vi "Init.vi"(5 "Bus In":refnum<class "Bus.lvclass">, 7 "Cluster":T1, 8 "error in (no error)":errorcluster, 9 "Init or Array":bool, 10 "Array":dbl[](array[numeric]), 11 "No-Op in":refnum<class "No-Op Output.lvclass">) -> (0 "error out":errorcluster, 2 "Bus Out":refnum<class "Bus.lvclass">, 3 "No-Op out":refnum<class "No-Op Output.lvclass">)   [LabVIEW 2024, in "No-Op Output.lvclass"]
uses:
  No-Op Output.lvclass
  Scaling/Scaling.lvclass
  Bus/Bus.lvclass
  No-Op Output.lvclass/No-Op Output.ctl
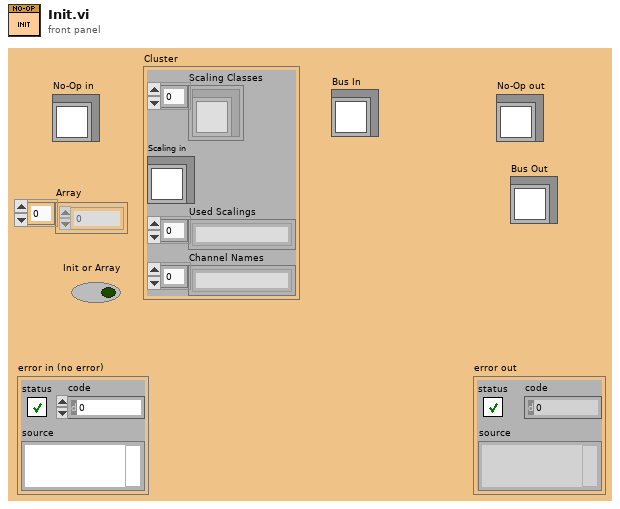
[diagram p1: front panel]
types:
  T1 = cluster{"Scaling Classes":refnum<class "Scaling.lvclass">[], "Scaling in":refnum<class "Scaling.lvclass">, "Used Scalings":string[], "Channel Names":string[]}
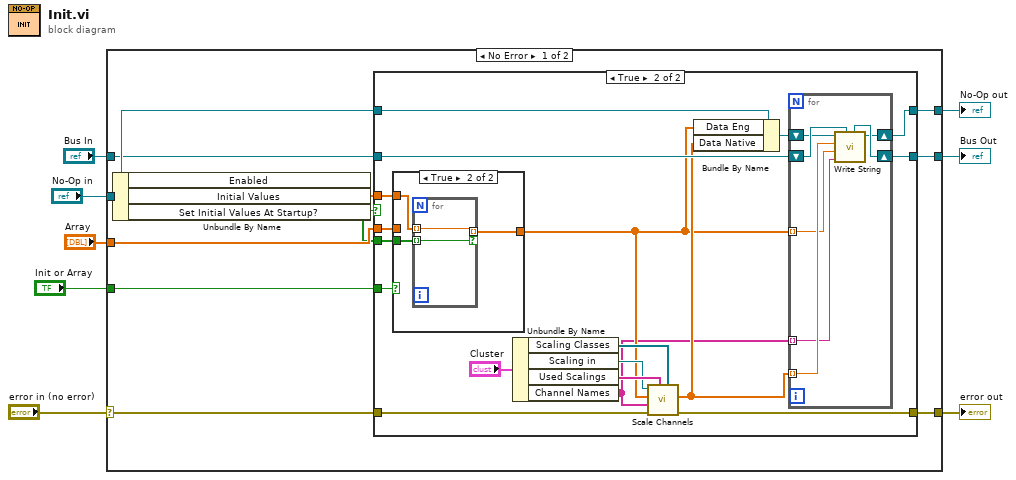
[diagram p0: block diagram]
diagram:
  n1 = case shown="No Error" "error in (no error)" {
    selector: "error in (no error)" -> [w16 w59]
    tunnel: [w15 w59] -> w7
    tunnel: [w12 w60] -> w6
    tunnel: "No-Op in" -> [w19 w60]
    tunnel: "Init or Array" -> [w18 _]
    tunnel: "Array" -> [w17 _]
    tunnel: "Bus In" -> [w14 w58]
    tunnel: [w13 w58] -> w1
    frame No Error {
      n2 = Unbundle By Name(w19) -> ("Enabled"=w11:bool[], "Initial Values"=w10:dbl[], "Set Initial Values At Startup?"=w9:bool)
      n3 = case shown="True" w9 {
        tunnel: w19 -> [w20 w40]
        tunnel: w18 -> [_ w39]
        tunnel: w17 -> [_ w38]
        tunnel: w16 -> [w22 w33]
        tunnel: [w22 w32] -> w15
        tunnel: w14 -> [w21 w31]
        tunnel: [w21 w30] -> w13
        tunnel: [w20 w29] -> w12
        tunnel: w11 -> [_ w24]
        tunnel: w10 -> [_ w23]
        frame False {
        }
        frame True {
          n4 = case shown="True" w39 {
            tunnel: w23 -> [_ w55]
            tunnel: [w48 w53] -> w26
            tunnel: w38 -> [w50 _]
            tunnel: w24 -> [w49 w54]
            frame False {
              n5 = for {
                tunnel: w50 -> [w52] mode=indexing
                tunnel: w49 -> [w51] mode=indexing
                tunnel: [w52] -> w48 mode=indexing if=w51
              }
            }
            frame True {
              n6 = for {
                tunnel: w55 -> [w57] mode=indexing
                tunnel: w54 -> [w56] mode=indexing
                tunnel: [w57] -> w53 mode=indexing if=w56
              }
            }
          }
          n7 = Unbundle By Name("Cluster") -> ("Scaling Classes"=w34:refnum<class "Scaling.lvclass">[], "Scaling in"=w36:refnum<class "Scaling.lvclass">, "Used Scalings"=w37:string[], "Channel Names"=w25:string[])
          n8 = call "Scale Channels.vi"("Scaling Classes"=w34, "Used Scalings"=w37, "error in (no error)"=w33, "Channel Names"=w25, "Values In"=w26, "Scaling in"=w36) -> ("error out"=w32:errorcluster, "Values Out"=w27:dbl[])  [unwired: 3 in, 1 out]
          n9 = Bundle By Name(cluster=w40, "Data Eng"=w26, "Data Native"=w27) -> (w28:refnum<class "No-Op Output.lvclass">)
          n10 = for {
            tunnel: w27 -> [w43] mode=indexing
            tunnel: w26 -> [w42] mode=indexing
            tunnel: w25 -> [w41] mode=indexing
            shift-right: [w46] -> w30
            shift-left: w31 -> [w47]
            shift-right: [w45] -> w29
            shift-left: w28 -> [w44]
            n11 = call-dynamic "Write String.vi"("Bus In"=w47, "Channel Name"=w41, "Data Value Engineering"=w42, "Data Value Native"=w43, "No-Op in"=w44) -> ("No-Op out"=w45:refnum<class "No-Op Output.lvclass">, "Bus Out"=w46:refnum<class "Bus.lvclass">)  [unwired: 4 in, 1 out]
          }
        }
      }
    }
    frame Error {
    }
  }
  "error out" <- w7
  "No-Op out" <- w6
  "Bus Out" <- w1
